vi "Main modul map v3 GPS + kinematyka.vi"() -> ()   [LabVIEW 2012]
uses:
  <vilib>/Utility/miscctls.llb/LVPoint32TypeDef.ctl
  <vilib>/Utility/miscctls.llb/LVBoundsTypeDef.ctl
  <vilib>/Utility/miscctls.llb/LVPointTypeDef.ctl
  Matematyczne/Matematyczne.lvlib
  <vilib>/addons/Fuzzy Logic/NI_Fuzzy_Logic_API.lvlib
  Pomocnicze/Pomocnicze.lvlib
panel:
  in  "Nowa Odl. od startu[m]":cluster{"X [m]":dbl, "Y [m]":dbl}={"X [m]"=-27.201483053257306, "Y [m]"=-30.40589390754667}
  out "x-y":u32
  in  "Lok. mapy odświeżanej":path=path "C:/Users/User/Desktop/Pliki moduł map off-line 2/auto.JPG"
  out "Prędkości kół":cluster{"prawe [rad/s]":dbl, "lewe [rad/s]":dbl}(graph)
  in  "Pocz. poł.":T1 {"UTM"."N [m]" format="%#_10g"}
  out "Mapa":picture caption="Mapa z wprowadzonym punktem"
  out "Lista współrzędnych":string[][](table)
  in  "Tab Control":T2(tab)
  in  "Azymut robota początkowy":dbl min=0.0 max=360.0
  in  "Lokalizacja mapy terenu":path=path "C:/Users/User/Desktop/pł.JPG"
  in  "Parametry odwzorowania Ziemi (WGS84)":cluster{"a":dbl, "b":dbl}={"a"=6378137.0, "b"=6356752.3142} {"b" format="%#.6g"; "a" format="%#.6g"}
  in  "Położenie na mapie":bool
  in  "Zakres skali":u16(ring)=11 items=["OSM 10m", "OSM 30m", "OSM 50m", "OSM 100m"]
  in  "Skalowanie":T3={"Polozenie 1"={"X"=265, "Y"=265}, "  Wybór \nznacznika"=FALSE, "   Polozenie 2"={"X"=358, "Y"=265}, "   Blokada \nznaczników"=FALSE, "Kolor  znaczników"=16774930, "Grubość \nznaczników"=2, "Wyznaczanie odległości"=enum."Odległość pomiędzy znacznikami", "Współrzędne geograficzne 1"="", "Współrzędne geograficzne 2"="", "Odl. pomiędzy znacznikami [m]"=15.0}
  in  "Zatwierdz ustalony zakres":bool
  in  "Odczyt GPS":bool
  in  "Obsługa punktów":T4 {"Usuń punkt z listy"."Punkt do usunięcia" items=["1"=1, "2"=2]}
  in  "Jazda":bool
  out "Dojazd do punktu":string
  out "Zatrzymanie \n w punkcie":bool
  in  "Położenie robota":bool
  in  "Położenie startu":bool
  in  "zad. promien odlegl.":dbl
  in  "Autonomia":bool
  out "Odległość\n od startu [m]":cluster{"X [m]":dbl, "Y [m]":dbl}
  out "Odczyt GPS":T5 caption="Aktualne położenie" {"Szerokośc geograficzna - GPS" format="%_9f"; "Długość geograficzna - GPS" format="%_9f"; "Położenie \nrobota  UTM"."E [m]" format="%#_10g"; "Położenie \nrobota  UTM"."N [m]" format="%#_12g"}
  in  "Właściwości mapy":T7={"Przesunięcie mapy"={"X"=0, "Y"=0}, "Dł. px[m]"=0.19634281539316645, "Zoom mapy"=1.0, "Wpisane punkty na\nliście współrzędnych"=12271, "Zaznaczony punkt"=15663118, "Układ współrzędnych"=0, "Kierunek ruchu robota"=15663118, "Początkowe położenie robota"=15663118, "Trasa robota"=0, "Ost. zazn. pkt"={"X"=0, "Y"=0}, "Draw Area Size"={"Width"=528, "Height"=564}} {"Zoom mapy" scale=0.2..4.0}
  in  "Mouse down":T8
  in  "stop":bool
  # "Ustawienia dla danych z GPS\nPodstaowe parametry Ziemi dla układu WGS84"
  # "Ustawienia dla kinematyki robota."
  # "Nie można usuwać \npunktów, gdy włączona \njest autonomia"
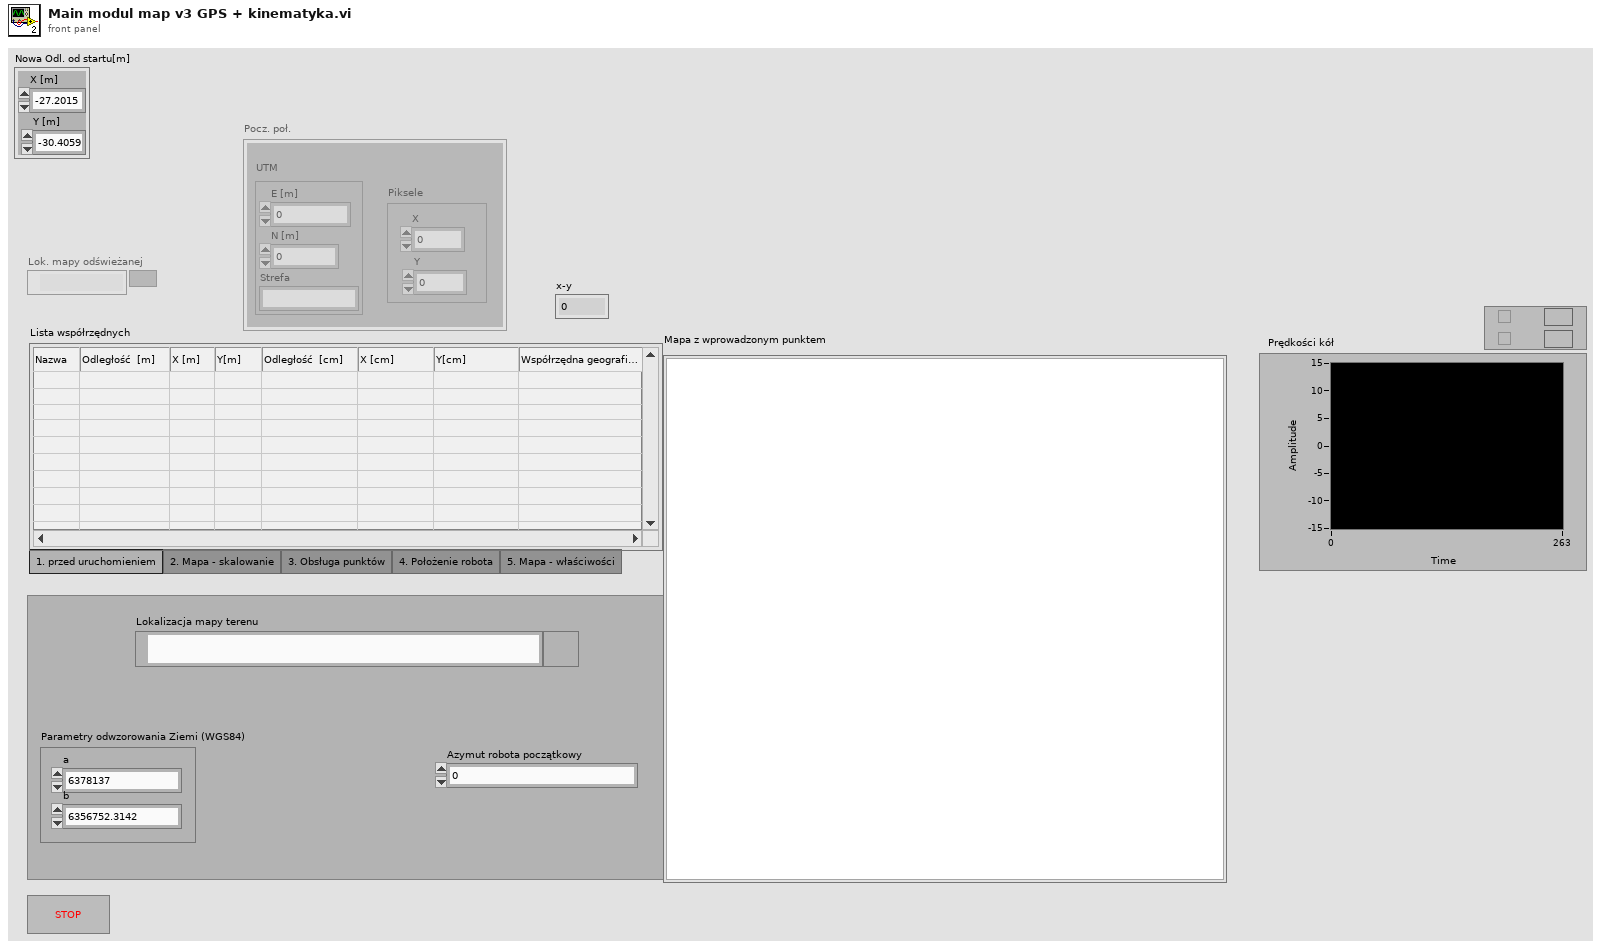
[diagram p1: front panel]
types:
  T1 = cluster{"UTM":cluster{"E [m]":ext, "N [m]":ext, "Strefa":string}, "Piksele":cluster{"X":i32, "Y":i32}}
  T2 = enum32{"1. przed uruchomieniem", "2. Mapa - skalowanie", "3. Obsługa punktów", "4. Położenie robota", "5. Mapa - właściwości"}
  T3 = cluster{"Polozenie 1":cluster{"X":i32, "Y":i32}, "  Wybór \nznacznika":bool, "   Polozenie 2":cluster{"X":i32, "Y":i32}, "   Blokada \nznaczników":bool, "Kolor  znaczników":u32, "Grubość \nznaczników":u32, "Wyznaczanie odległości":enum16{"Współrzędne geograficzne", "Odległość pomiędzy znacznikami"}, "Współrzędne geograficzne 1":string, "Współrzędne geograficzne 2":string, "Odl. pomiędzy znacznikami [m]":dbl}
  T4 = cluster{"Zaznaczony punkt":cluster{"Nazwa":string, "Odl. do pkt [m]":cluster{"X":dbl, "Y":dbl}, "Dodaj punkt odl.":bool}, "Wsp. geograficzne":cluster{"Nazwa":string, "Współrzędna punktu":string, "Dodaj punkt wsp.":bool}, "Usuń punkt z listy":cluster{"Punkt do usunięcia":u16, "Usuń punkt":bool}}
  T5 = cluster{"Położenie \nrobota  UTM":cluster{"E [m]":ext, "N [m]":ext, "Strefa":string}, "Długość geograficzna - GPS":dbl, "Szerokośc geograficzna - GPS":dbl, "Azymut [stopnie]":dbl}
  T6 = typedef "LVBoundsTypeDef.ctl" = cluster{"Width":u32, "Height":u32}
  T7 = cluster{"Przesunięcie mapy":cluster{"X":i16, "Y":i16}, "Dł. px[m]":dbl, "Zoom mapy":sgl, "Wpisane punkty na\nliście współrzędnych":u32, "Zaznaczony punkt":u32, "Układ współrzędnych":u32, "Kierunek ruchu robota":u32, "Początkowe położenie robota":u32, "Trasa robota":u32, "Ost. zazn. pkt":cluster{"X":i32, "Y":i32}, "Draw Area Size":T6}
  T8 = typedef "LVPoint32TypeDef.ctl" = cluster{"Horizontal":i32, "Vertical":i32}
  T9 = enum16{"Pobranie punktu", "Obrót i dojazd do punktu", "Zatrzymanie w punkcie"}
  T10 = typedef "NI_Fuzzy_Logic_API.lvlib/FL System.ctl" = cluster{"input variables":T11[], "output variables":T11[], "rules":T14[], "defuzzification method":T20, "description":string, "user MF interpolating polynomials":T21[]}
  T11 = typedef "NI_Fuzzy_Logic_API.lvlib/FL Variable.ctl" = cluster{"name":string, "range":dbl[], "MFs":T12[]}
  T12 = typedef "NI_Fuzzy_Logic_API.lvlib/FL Membership Function.ctl" = cluster{"name":string, "shape":T13, "points":dbl[], "color":u32, "user-defined shape index":i32}
  T13 = typedef "NI_Fuzzy_Logic_API.lvlib/FL Membership Function Shape.ctl" = u16
  T14 = typedef "NI_Fuzzy_Logic_API.lvlib/FL Rule.ctl" = cluster{"antecedents":T15[], "antecedent connective":T17, "consequents":T18[], "consequent implication":T19, "degree of support":dbl}
  T15 = typedef "NI_Fuzzy_Logic_API.lvlib/FL Antecedent.ctl" = cluster{"Var Index":i32, "MF Index":i32, "Cond":T16}
  T16 = typedef "NI_Fuzzy_Logic_API.lvlib/FL Modifier.ctl" = u16
  T17 = typedef "NI_Fuzzy_Logic_API.lvlib/FL Antecedent Connective.ctl" = u16
  T18 = typedef "NI_Fuzzy_Logic_API.lvlib/FL Consequent.ctl" = cluster{"Var Index":i32, "MF Index":i32, "Cond":T16}
  T19 = typedef "NI_Fuzzy_Logic_API.lvlib/FL Consequent Implication.ctl" = u16
  T20 = typedef "NI_Fuzzy_Logic_API.lvlib/FL Defuzzification.ctl" = u16
  T21 = typedef "NI_Fuzzy_Logic_API.lvlib/FL Interpolating polynomials.ctl" = cluster{"X":dbl[], "Y":dbl[], "Y(x) coeff":dbl[][], "X(y) coeff":dbl[][], "Area(y) coeff":dbl[][], "coa_x(y) coeff":dbl[][]}
  T22 = cluster{"left":i16, "top":i16, "right":i16, "bottom":i16}
  T23 = cluster{"Odl. robota od startu [m]":cluster{"X":dbl, "Y":dbl}, "Położenie startowe":cluster{"X":i32, "Y":i32}, "Azymut [stopnie]":dbl}
  T24 = cluster{"Rozmiar mapy":cluster{"Szerokość":i16, "Wysokość":i16}, "Dł. piksela [m]":dbl, "Trasa robota":u32, "Poł. startowe\n piksele":cluster{"X":i32, "Y":i32}}
  T25 = cluster{"Położenie":cluster{"Pixel x":i16, "Pixel y":i16}, "Kolor punktu":u32, "Rozmiar punktu":u32, "Nazwa punktu":string}
  T26 = cluster{"Kolor punktów z listy":u32, "Położenie startowe robota":cluster{"Pixel y":i16, "Pixel x":i16}}
  T27 = typedef "LVPointTypeDef.ctl" = cluster{"Horizontal":i16, "Vertical":i16}
  T28 = cluster{"Przesunięcie mapy":cluster{"X":i16, "Y":i16}, "Długość piksela w metrach":dbl, "Zoom mapy":sgl, "Wpisane punkty na\nliście współrzędnych":u32, "Zaznaczony punkt":u32, "Układ współrzędnych":u32, "Kierunek ruchu robota":u32, "Początkowe położenie robota":u32, "Trasa robota":u32, "Ostatni zaznaczony punkt na mapie":cluster{"X":i32, "Y":i32}, "Draw Area Size":T6}
  T29 = typedef "LVMouseTypeDef.ctl" = cluster{"Mouse Position":cluster{"X":i32, "Y":i32}, "Mouse Modifiers":cluster{"Button Down":bool, "Shift Mod":bool, "Menu Mod":bool, "Option Mod":bool}}
  T30 = cluster{"Przesunięcie mapy":cluster{"X":i16, "Y":i16}, "Długość piksela w metrach":dbl, "Zoom mapy":sgl, "Wpisane punkty na\nliście współrzędnych":u32, "Zaznaczony punkt":u32, "Układ współrzędnych":u32, "Kierunek ruchu robota":u32, "Początkowe położenie robota":u32, "Trasa robota":u32, "Ost. zazn. pkt.":cluster{"X":i32, "Y":i32}, "Draw Area Size":T6}
  T31 = cluster{"Zaznaczony punkt":cluster{"Nazwa":string, "Odleglosc do\n zaznaczonego punktu [m]":cluster{"X":dbl, "Y":dbl}, "Dodaj punkt odl.":bool}, "Wsp. geograficzne":cluster{"Nazwa":string, "Współrzędna punktu":string, "Dodaj punkt wsp.":bool}, "Usuń punkt z listy":cluster{"Punkt do usunięcia":u16, "Usuń punkt":bool}}
  T32 = cluster{"E [m]":ext, "N [m]":ext, "Strefa":string}
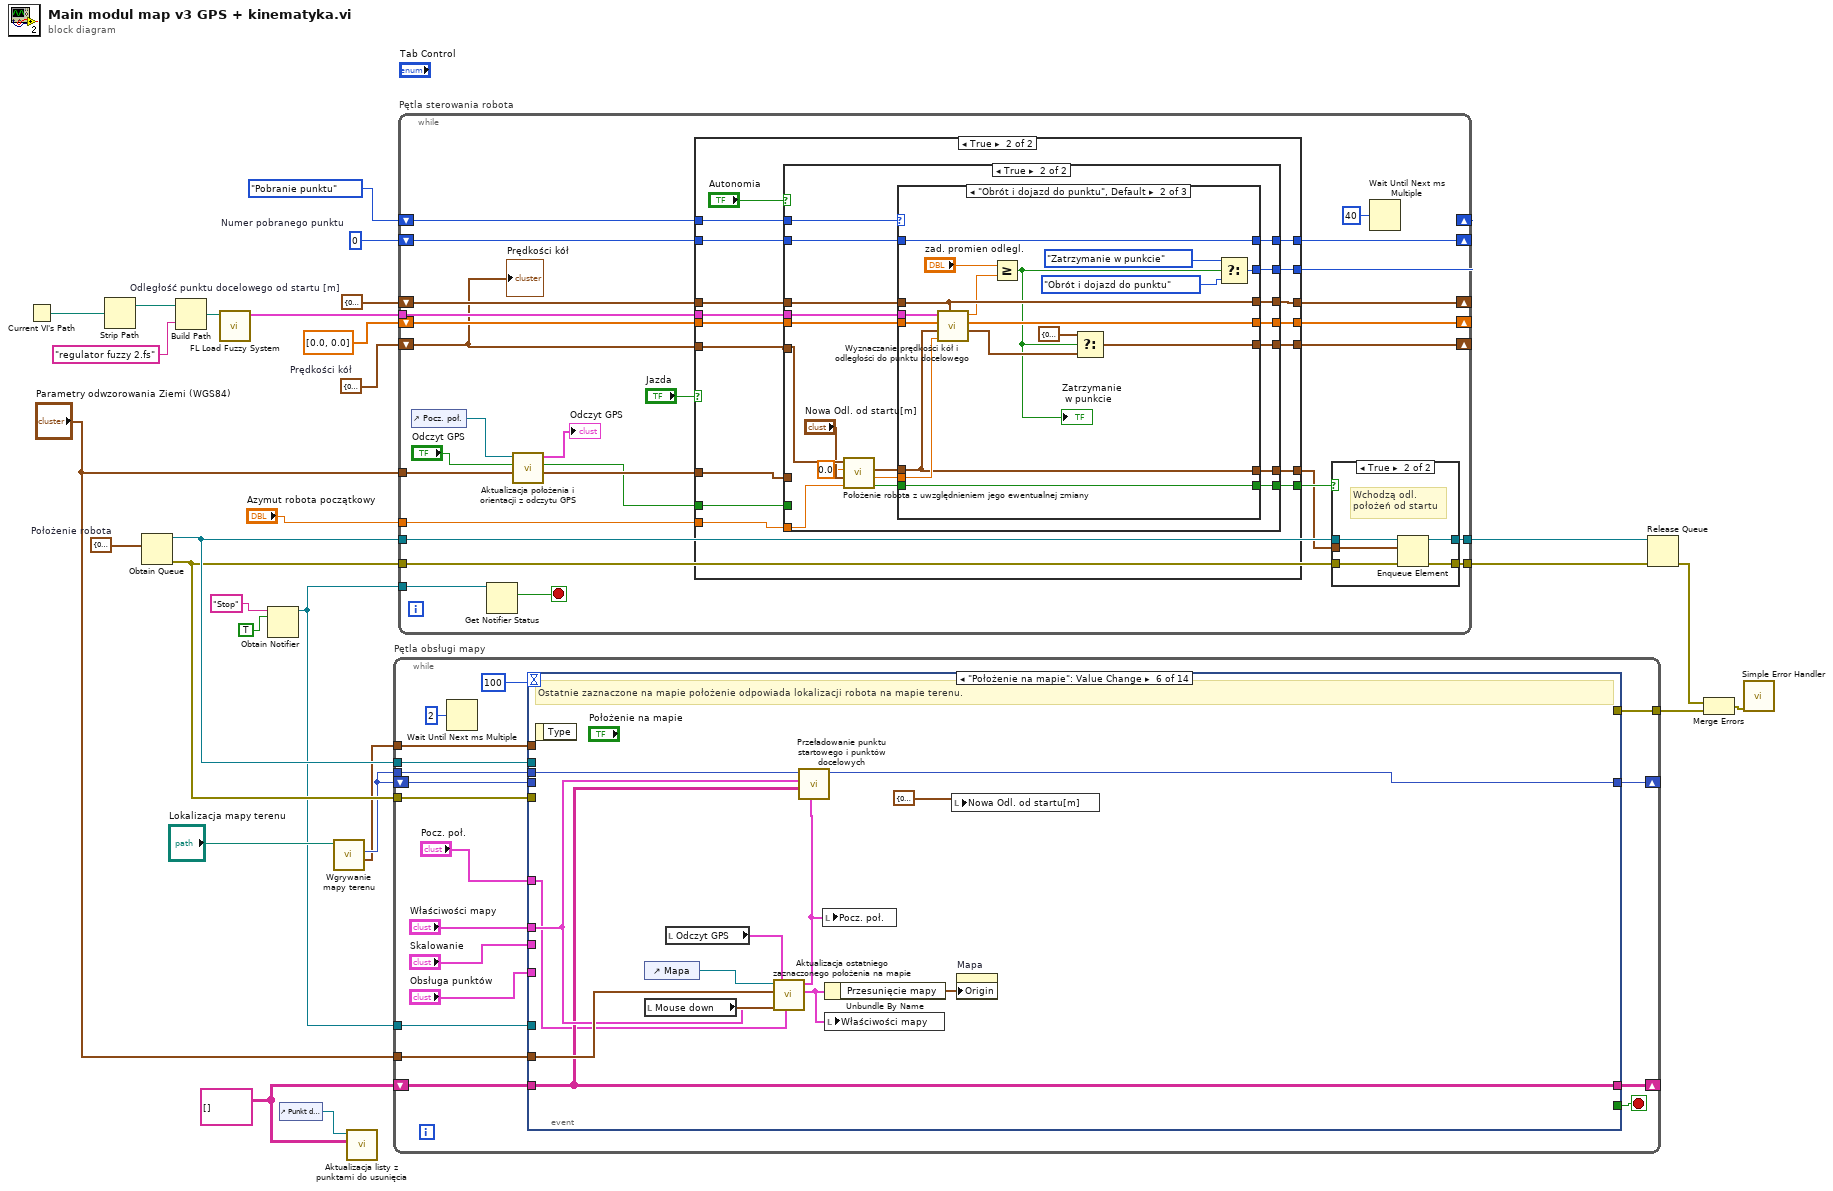
[diagram p0: block diagram]
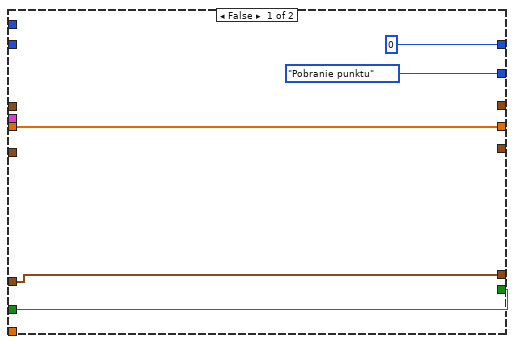
[diagram p3: hidden frame]
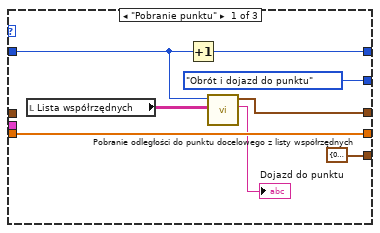
[diagram p4: hidden frame]
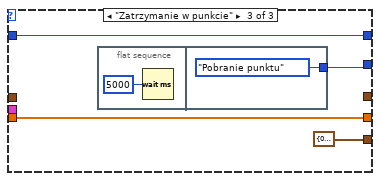
[diagram p5: hidden frame]
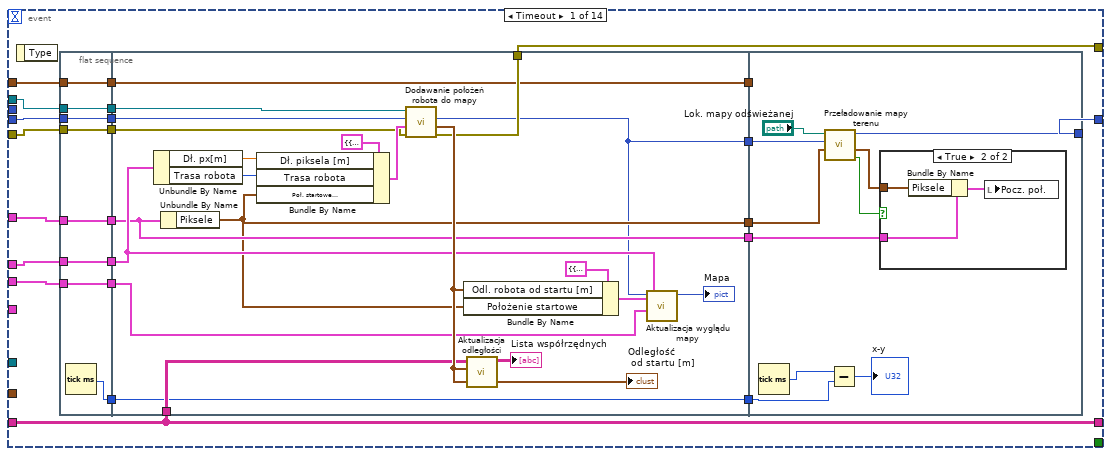
[diagram p7: hidden frame]
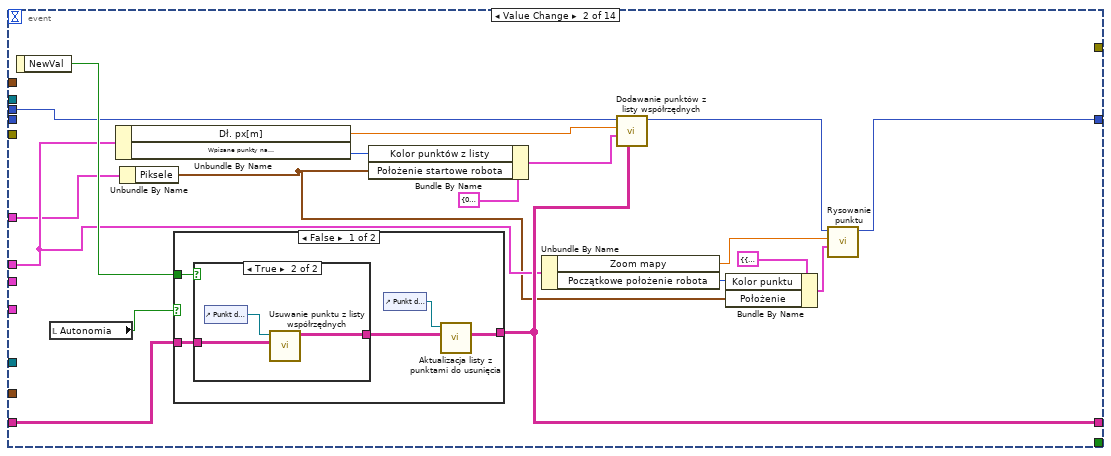
[diagram p9: hidden frame]
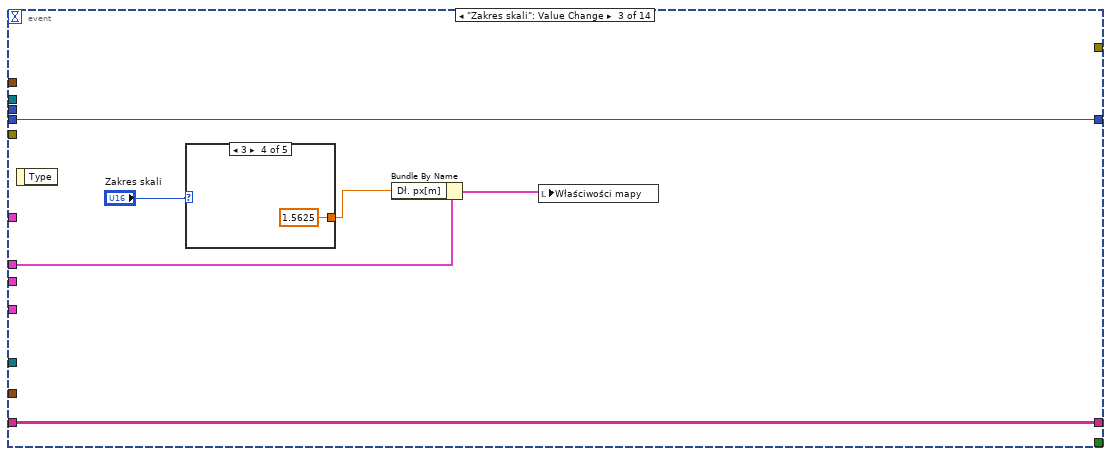
[diagram p12: hidden frame]
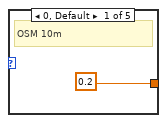
[diagram p13: hidden frame]
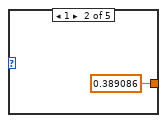
[diagram p14: hidden frame]
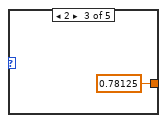
[diagram p15: hidden frame]
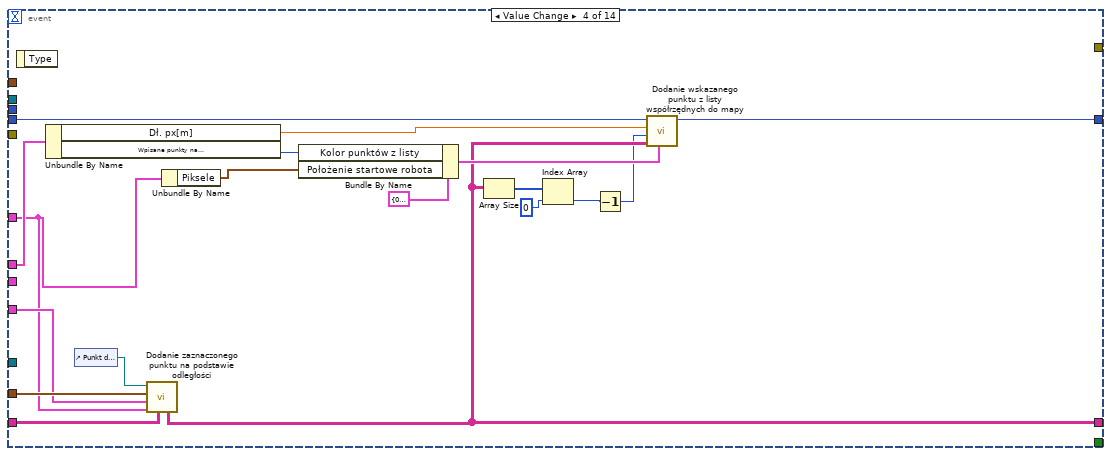
[diagram p17: hidden frame]
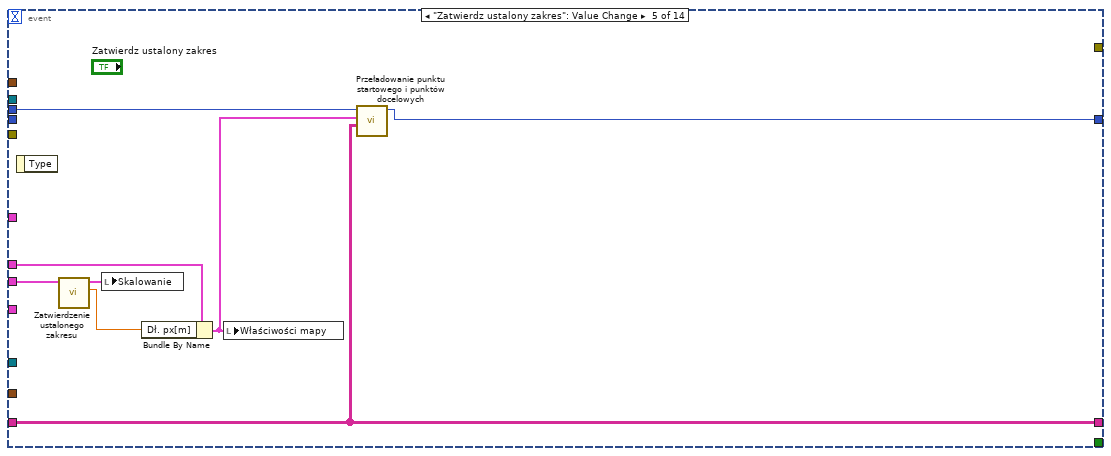
[diagram p18: hidden frame]
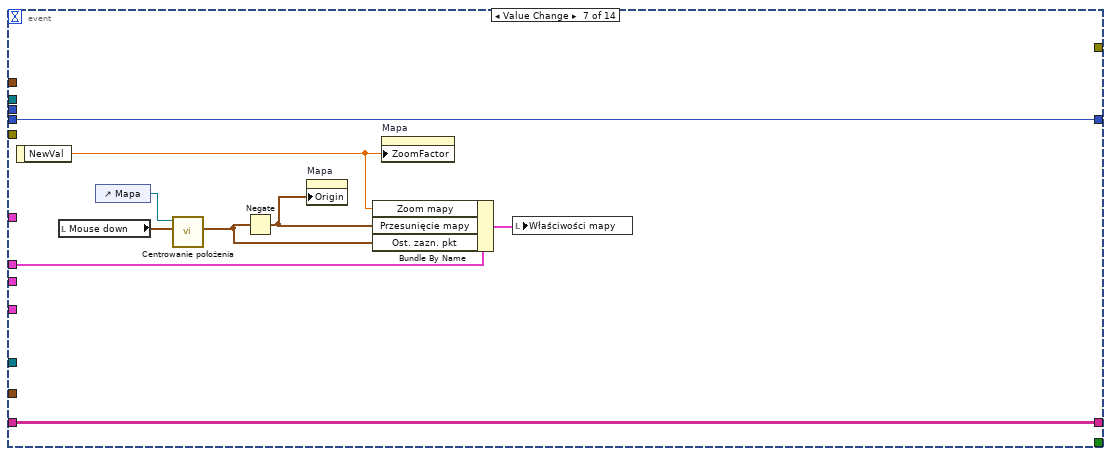
[diagram p19: hidden frame]
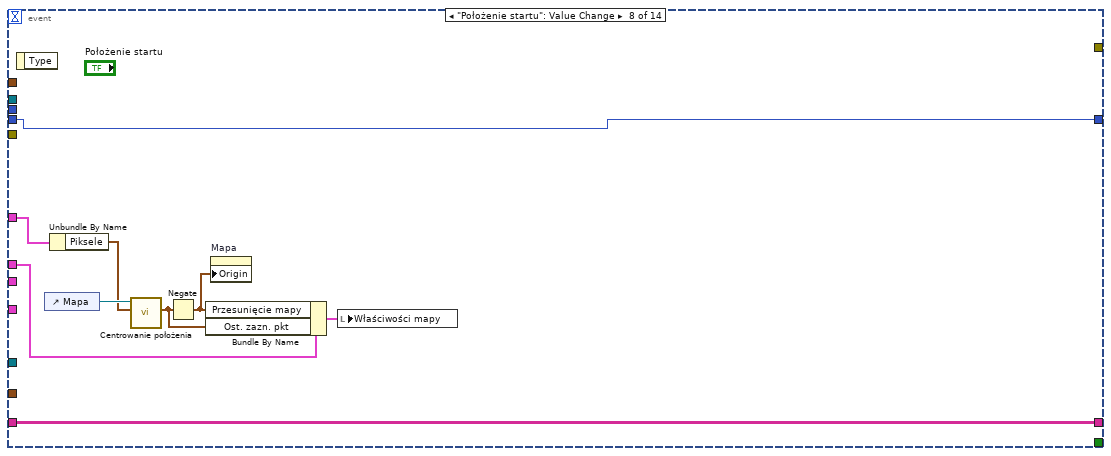
[diagram p20: hidden frame]
diagram:
  w6 = cluster{"prawe [rad/s]":dbl, "lewe [rad/s]":dbl} {"prawe [rad/s]"=0.0, "lewe [rad/s]"=0.0}  # Prędkości kół
  w13 = cluster{"X [m]":dbl, "Y [m]":dbl} {"X [m]"=0.0, "Y [m]"=0.0}  # Położenie robota
  w28 = string[][] [] ("Lista współrzędnych")
  w18 = cluster{"X/E [m]":dbl, "Y/N [m]":dbl} {"X/E [m]"=0.0, "Y/N [m]"=0.0}  # Odległość punktu docelowego od startu [m]
  w19 = 0  # Numer pobranego punktu
  n1 = Current VI's Path() -> (path=w25:path)
  n2 = Strip Path(path=w25) -> (stripped path=w23:path)  [unwired: 1 out]
  n3 = Obtain Queue(element data type=w13) -> (queue out=w10:refnum<queue>, error out=w9:errorcluster)  [unwired: 4 in, 1 out]
  n4 = Build Path(base path=w23, name or relative path="regulator fuzzy 2.fs") -> (appended path=w22:path)
  n5 = call <vilib>:"FL Load Fuzzy System.vi"("file path"=w22) -> ("fuzzy system out"=w21:T10)  [unwired: 1 in, 9 out]
  n6 = Obtain Notifier(name (unnamed)="Stop", notification data type=TRUE ("create if not found? (T)")) -> (notifier out=w4:refnum<notifier>)  [unwired: 2 in, 2 out]
  n7 = control-ref of="Punkt do usunięcia"() -> (w15:refnum<vi>)
  n8 = call "Wgrywanie mapy terenu.vi"("Lokalizacja mapy terenu"="Lokalizacja mapy terenu") -> ("Rozmiar mapy"=w2:T22, "Mapa terenu"=w5:picture)  [unwired: 9 in]
  n9 = call "Aktualizacja listy z punktami do usunięcia.vi"("Lista współrzędnych"=w28, "Lista z punktami do usunięcia"=w15) -> ()  [unwired: 10 in]
  n10 = while "Pętla obsługi mapy" {
    shift-right: [w43] -> _
    shift-left: w5 -> [w44]
    shift-right: [w41] -> _
    shift-left: w28 -> [w42]
    tunnel: "Parametry odwzorowania Ziemi (WGS84)" -> [w40]
    tunnel: w4 -> [w39]
    tunnel: w10 -> [w38]
    tunnel: w9 -> [w33]
    tunnel: w5 -> [w32]
    tunnel: [w31] -> w3
    tunnel: w2 -> [w30]
    stop <- w46 stop-if-true
    n11 = Wait Until Next ms Multiple(millisecond multiple=u32 2) -> ()  [unwired: 1 out]
    n12 = event shown="[5] \"Położenie na mapie\": Value Change" {
      selector: _ -> [_ _ _ _ _ _ _ _ _ _ _ _ _ _]
      dyn-events: _ -> [_ _ _ _ _ _ _ _ _ _ _ _ _ _]
      timeout: 100 -> [_ _ _ _ _ _ _ _ _ _ _ _ _ _]
      tunnel: "Właściwości mapy" -> [w68 w115 w141 w161 w171 w180 w189 w201 w212 w228 _ w247 w267 w286]
      tunnel: w44 -> [w65 _ w144 w154 _ _ w196 w198 w218 w231 w235 w249 w275 w280]
      tunnel: [_ _ _ _ _ _ _ _ _ "stop" _ _ _ _] -> w46
      tunnel: [w61 w113 w144 w150 w167 w178 w196 w198 w218 w231 w235 w249 w275 w277] -> w43
      tunnel: w42 -> [w66 w128 w143 w163 w168 w179 w195 w199 w217 w230 w234 w248 w274 w295]
      tunnel: [w66 w122 w143 w155 w168 w179 w195 w199 w217 w230 w234 w248 w274 w283] -> w41
      tunnel: w40 -> [_ _ _ w166 _ w186 _ _ _ _ _ _ _ _]
      tunnel: w39 -> [_ _ _ _ _ _ _ _ _ w229 _ _ _ _]
      tunnel: w38 -> [w64 _ _ _ _ _ _ _ _ _ _ _ _ _]
      tunnel: "Pocz. poł." -> [w58 w112 _ w149 _ w176 _ w197 w206 _ _ w236 w260 w276]
      tunnel: "Skalowanie" -> [w67 _ _ _ w174 _ _ _ _ _ _ w238 _ _]
      tunnel: "Obsługa punktów" -> [_ _ _ w164 _ _ _ _ _ _ _ w245 w263 w290]
      tunnel: w33 -> [w63 _ _ _ _ _ _ _ _ _ _ _ _ _]
      tunnel: w32 -> [_ w125 _ _ w170 w181 _ _ _ _ _ _ _ _]
      tunnel: [w62 _ _ _ _ _ _ _ _ _ _ _ _ _] -> w31
      tunnel: w30 -> [w59 _ _ _ _ _ _ _ _ _ _ _ _ _]
      event Timeout {
        n13 = event-data() -> ()  [unwired: 1 in, 1 out]
        n14 = flat-sequence {
          tunnel: w58 -> [w71]
          tunnel: w59 -> [w72]
          tunnel: w63 -> [w73]
          tunnel: w64 -> [w74]
          tunnel: w65 -> [w75]
          tunnel: w67 -> [w76]
          tunnel: w68 -> [w77]
          tunnel: [w77] -> w55
          tunnel: [w76] -> w54
          tunnel: [w75] -> w53
          tunnel: [w74] -> w52
          tunnel: [w73] -> w51
          tunnel: [w72] -> w50
          tunnel: [w71] -> w49
          tunnel: [w70] -> w48
          tunnel: [w79] -> w69
          tunnel: w66 -> [w88]
          tunnel: [w84] -> w62
          tunnel: [w83] -> w60
          tunnel: [w80] -> w57
          tunnel: [w81] -> w56
          tunnel: w55 -> [w82]
          tunnel: w54 -> [w89]
          tunnel: w53 -> [w87]
          tunnel: w52 -> [w86]
          tunnel: w51 -> [w85]
          tunnel: w50 -> [w83]
          tunnel: w49 -> [w81]
          tunnel: w48 -> [w78]
          tunnel: [w78] -> w47
          tunnel: [w108] -> w61
          tunnel: w69 -> [w107]
          tunnel: w60 -> [_]
          tunnel: w57 -> [w106]
          tunnel: w56 -> [w102]
          tunnel: w47 -> [w100]
          frame #0 {
            n15 = Tick Count (ms)() -> (millisecond timer value=w70:u32)
          }
          frame #1 {
            n16 = Unbundle By Name(w82) -> ("Dł. px[m]"=w94:dbl, "Trasa robota"=w95:u32)
            n17 = Unbundle By Name(w81) -> ("Piksele"=w80:cluster{"X":i32, "Y":i32})
            n18 = Bundle By Name(cluster=T24 {"Rozmiar mapy"={"Szerokość"=0, "Wysokość"=0}, "Dł. piksela [m]"=0.19634281539316645, "Trasa robota"=16722479, "Poł. startowe\n piksele"={"X"=0, "Y"=0}} ("Dane do wyzn. poł. robota na mapie 2"), "Dł. piksela [m]"=w94, "Trasa robota"=w95, "Poł. startowe\n piksele"=w80) -> (w98:T24)
            n19 = call "Dodawanie położeń robota do mapy.vi"("error in (no error)"=w85, "Dane do wyzn. poł. robota na mapie"=w98, "Mapa terenu"=w87, "Dane z położenia"=w86) -> ("error out"=w84:errorcluster, "Odległość robota od startu [m]"=w97:cluster{"X [m]":dbl, "Y [m]":dbl}, "Mapa z wprowadzonym punktem"=w79:picture)  [unwired: 5 in]
            "Odległość\n od startu [m]" <- w97
            n20 = Bundle By Name(cluster=T23 {"Odl. robota od startu [m]"={"X"=246.0, "Y"=243.0}, "Położenie startowe"={"X"=246, "Y"=243}, "Azymut [stopnie]"=297.94899101038743} ("Położenie robota"), "Odl. robota od startu [m]"=w97, "Położenie startowe"=w80) -> (w96:T23)
            n21 = call "Aktualizacja odległości.vi"("Odległość od startu [m]"=w97, "Lista współrzędnych"=w88) -> ("Lista współrzędnych 2"=→"Lista współrzędnych":string[][])  [unwired: 9 in]
            n22 = call "Aktualizacja wyglądu mapy.vi"("Położenie robota"=w96, "Skalowanie i kolory"=w89, "Właściwości mapy"=w82, "Mapa"=w79) -> ("Przesunięta mapa"=→"Mapa":picture)  [unwired: 7 in]
          }
          frame #2 {
            n23 = Tick Count (ms)() -> (millisecond timer value=w101:u32)
            n24 = call "Przeładowanie mapy terenu.vi"("Położenie startowe"=w106, ">mapa z trasą robota>"=w107, "path to JPEG file"="Lok. mapy odświeżanej") -> ("reload"=w105:bool, "Nowe położenie  startowe [px]"=w103:cluster{"X [px]":i16, "Y [px]":i16}, "Mapa terenu"=w108:picture)  [unwired: 6 in]
            n25 = Subtract(x=w101, y=w100) -> (x-y=→"x-y":u32)
            n26 = case shown="True" w105 {
              tunnel: w103 -> [_ w111]
              tunnel: w102 -> [_ w110]
              frame False {
              }
              frame True {
                n27 = Bundle By Name(cluster=w110, "Piksele"=w111) -> (w109:T1)
                n28 = local write "Pocz. poł."(w109) -> ()
              }
            }
          }
        }
      }
      event "Obsługa punktów.Usuń punkt z listy.Usuń punkt": Value Change {
        n29 = event-data() -> ("NewVal"=w129:bool)  [unwired: 1 in]
        n30 = local read "Autonomia"() -> (w127:bool)
        n31 = Unbundle By Name(w115) -> ("Dł. px[m]"=w124:dbl, "Wpisane punkty na\nliście współrzędnych"=w126:u32)
        n32 = Unbundle By Name(w112) -> ("Piksele"=w114:cluster{"X":i32, "Y":i32})
        n33 = case shown="False" w127 {
          tunnel: w129 -> [w133 _]
          tunnel: w128 -> [w131 w138]
          tunnel: [w130 w138] -> w122
          frame False {
            n34 = case shown="True" w133 {
              tunnel: w131 -> [w134 w136]
              tunnel: [w134 w135] -> w130
              frame False {
              }
              frame True {
                n35 = control-ref of="Punkt do usunięcia"() -> (w137:refnum<vi>)
                n36 = call "Usuwanie punktu z listy współrzędnych.vi"("Lista współrzędnych"=w136, "Lista z punktami do usunięcia"=w137) -> ("Lista współrzędnych 2"=w135:string[][])  [unwired: 9 in]
              }
            }
            n37 = control-ref of="Punkt do usunięcia"() -> (w132:refnum<vi>)
            n38 = call "Aktualizacja listy z punktami do usunięcia.vi"("Lista współrzędnych"=w130, "Lista z punktami do usunięcia"=w132) -> ()  [unwired: 10 in]
          }
          frame True {
          }
        }
        n39 = Bundle By Name(cluster=T26 {"Kolor punktów z listy"=0, "Położenie startowe robota"={"Pixel y"=0, "Pixel x"=0}} ("Właściwości punktów z listy"), "Kolor punktów z listy"=w126, "Położenie startowe robota"=w114) -> (w121:T26)
        n40 = Unbundle By Name(w115) -> ("Zoom mapy"=w118:sgl, "Początkowe położenie robota"=w117:u32)
        n41 = call "Dodawanie punktów z listy współrzędnych.vi"("Lista współrzędnych"=w122, "Właściwości punktów z listy"=w121, "Długość piksela w metrach"=w124, "Mapa terenu"=w125) -> ("Mapa z wprowadzonym punktem"=w116:picture)  [unwired: 6 in, 1 out]
        n42 = Bundle By Name(cluster=T25 {"Położenie"={"Pixel x"=246, "Pixel y"=243}, "Kolor punktu"=15663118, "Rozmiar punktu"=2, "Nazwa punktu"=""} ("Punkt na mapie"), "Kolor punktu"=w117, "Położenie"=w114) -> (w119:T25)
        n43 = call "Rysowanie punktu.vi"("Punkt na mapie"=w119, "Zoom mapy"=w118, "Mapa terenu"=w116) -> ("Mapa z wprowadzonym punktem"=w113:picture)  [unwired: 8 in]
      }
      event "Zakres skali": Value Change {
        n44 = event-data() -> ()  [unwired: 1 in, 1 out]
        n45 = case shown="3" "Zakres skali" {
          tunnel: [0.2 0.389086 0.78125 1.5625 _] -> w139
          frame 0, Default {
            # "OSM 10m"
          }
          frame 1 {
          }
          frame 2 {
          }
          frame 3 {
          }
          frame 4 {
          }
        }
        n46 = Bundle By Name(cluster=w141, "Dł. px[m]"=w139) -> (w140:T7)
        n47 = local write "Właściwości mapy"(w140) -> ()
      }
      event "Obsługa punktów.Zaznaczony punkt.Dodaj punkt odl.": Value Change {
        n48 = event-data() -> ()  [unwired: 1 in, 1 out]
        n49 = Unbundle By Name(w161) -> ("Dł. px[m]"=w157:dbl, "Wpisane punkty na\nliście współrzędnych"=w160:u32)
        n50 = control-ref of="Punkt do usunięcia"() -> (w165:refnum<vi>)
        n51 = call "Dodanie zaznaczonego punktu na podstawie odległości.vi"("output array in"=w163, "Pocz. poł."=w149, "Obsługa punktów"=w164, "Parametry odwzorowania Ziemi (WGS84)"=w166, "Ring in"=w165) -> ("output array out"=w155:string[][])  [unwired: 6 in]
        n52 = Unbundle By Name(w149) -> ("Piksele"=w151:cluster{"X":i32, "Y":i32})
        n53 = Bundle By Name(cluster=T26 {"Kolor punktów z listy"=0, "Położenie startowe robota"={"Pixel y"=0, "Pixel x"=0}} ("Właściwości punktów z listy"), "Kolor punktów z listy"=w160, "Położenie startowe robota"=w151) -> (w156:T26)
        n54 = Array Size(array=w155) -> (size(s)=w158:i32[])
        n55 = Index Array(array=w158, index=0) -> (element=w153:i32)
        n56 = Decrement(x=w153) -> (x-1=w152:i32)
        n57 = call "Dodanie wskazanego punktu z listy współrzędnych do mapy.vi"("Właściwości punktów z listy"=w156, "Lista współrzędnych"=w155, "Nr punktu"=w152, "Długość piksela w metrach"=w157, "Mapa terenu"=w154) -> ("Mapa z wprowadzonym punktem"=w150:picture)  [unwired: 5 in, 1 out]
      }
      event "Zatwierdz ustalony zakres": Value Change {
        n58 = event-data() -> ()  [unwired: 1 in, 1 out]
        n59 = call "Zatwierdzenie ustalonego zakresu.vi"("Skalowanie in"=w174) -> ("Dł. piksela[m]"=w172:dbl, "Skalowanie out"=w173:T3)  [unwired: 9 in]
        n60 = local write "Skalowanie"(w173) -> ()
        n61 = Bundle By Name(cluster=w171, "Dł. px[m]"=w172) -> (w169:T7)
        n62 = local write "Właściwości mapy"(w169) -> ()
        n63 = call "Przeładowanie punktu startowego i punktów docelowych.vi"("Lista współrzędnych"=w168, "Właściwości mapy"=w169, "Mapa terenu"=w170) -> ("Mapa z wprowadzonym punktem"=w167:picture)  [unwired: 8 in]
      }
      event "Położenie na mapie": Value Change {
        # "Ostatnie zaznaczone na mapie położenie odpowiada lokalizacji robota na mapie terenu."
        n64 = event-data() -> ()  [unwired: 1 in, 1 out]
        n65 = control-ref of="Mapa"() -> (w185:refnum<vi>)
        n66 = local read "Mouse down"() -> (w187:T8)
        n67 = local read "Odczyt GPS"() -> (w182:T5)
        n68 = call "Aktualizacja ostatniego zaznaczonego położenia na mapie.vi"("Pocz. poł."=w176, "Aktualne położenie"=w182, "Właściwości mapy in"=w180, "Mouse down coords"=w187, "Parametry odwzorowania Ziemi (WGS84)"=w186, "Picture in"=w185) -> ("Właściwości mapy out"=w184:T28, "Pocz. poł. 2"=w177:T1)  [unwired: 4 in]
        n69 = call "Przeładowanie punktu startowego i punktów docelowych.vi"("Pocz. poł. in"=w177, "Lista współrzędnych"=w179, "Właściwości mapy"=w180, "Mapa terenu"=w181) -> ("Mapa z wprowadzonym punktem"=w178:picture)  [unwired: 7 in]
        n70 = local write "Pocz. poł."(w177) -> ()
        n71 = Unbundle By Name(w184) -> ("Przesunięcie mapy"=w183:cluster{"X":i16, "Y":i16})
        n72 = local write "Właściwości mapy"(w184) -> ()
        n73 = local write "Nowa Odl. od startu[m]"(cluster{"X [m]":dbl, "Y [m]":dbl} {"X [m]"=0.0, "Y [m]"=0.0} ("Nowa Odl. od startu[m]")) -> ()
        n74 = property on="Mapa" class="Pict"("Origin"=w183) -> ()  [unwired: 2 in, 2 out]
      }
      event "Właściwości mapy.Zoom mapy": Value Change {
        n75 = event-data() -> ("NewVal"=w193:sgl)  [unwired: 1 in]
        n76 = local read "Mouse down"() -> (w188:T8)
        n77 = control-ref of="Mapa"() -> (w194:refnum<vi>)
        n78 = call "Centrowanie położenia.vi"("Ostatnie położenie robota"=w188, "Mapa z wprowadzonym punktem"=w194) -> ("Przesunięcie wycentrowane"=w191:T8)  [unwired: 9 in]
        n79 = Negate(x=w191) -> (-x=w190:T8)
        n80 = property on="Mapa" class="Pict"("Origin"=w190) -> ()  [unwired: 2 in, 2 out]
        n81 = Bundle By Name(cluster=w189, "Zoom mapy"=w193, "Przesunięcie mapy"=w190, "Ost. zazn. pkt"=w191) -> (w192:T7)
        n82 = property on="Mapa" class="Pict"("ZoomFactor"=w193) -> ()  [unwired: 2 in, 2 out]
        n83 = local write "Właściwości mapy"(w192) -> ()
      }
      event "Położenie startu": Value Change {
        n84 = event-data() -> ()  [unwired: 1 in, 1 out]
        n85 = control-ref of="Mapa"() -> (w205:refnum<vi>)
        n86 = Unbundle By Name(w197) -> ("Piksele"=w200:cluster{"X":i32, "Y":i32})
        n87 = call "Centrowanie położenia.vi"("Ostatnie położenie robota"=w200, "Mapa z wprowadzonym punktem"=w205) -> ("Przesunięcie wycentrowane"=w203:T8)  [unwired: 9 in]
        n88 = Negate(x=w203) -> (-x=w202:T8)
        n89 = Bundle By Name(cluster=w201, "Przesunięcie mapy"=w202, "Ost. zazn. pkt"=w203) -> (w204:T7)
        n90 = property on="Mapa" class="Pict"("Origin"=w202) -> ()  [unwired: 2 in, 2 out]
        n91 = local write "Właściwości mapy"(w204) -> ()
      }
      event "Położenie robota": Value Change {
        n92 = event-data() -> ()  [unwired: 1 in, 1 out]
        n93 = local read "Odległość\n od startu [m]"() -> (w211:cluster{"X [m]":dbl, "Y [m]":dbl})
        n94 = Unbundle By Name(w212) -> ("Dł. px[m]"=w210:dbl)
        n95 = Unbundle By Name(w206) -> ("Piksele"=w208:cluster{"X":i32, "Y":i32})
        n96 = in-place {
          in-place-border: w210 -> [w221]
          n97 = in-place-cluster #1(w211) -> ("X [m]"=w220:dbl, "Y [m]"=w219:dbl)
          n98 = Divide(x=w219, y=w221) -> (x/y=w222:dbl)
          n99 = Divide(x=w220, y=w221) -> (x/y=w224:dbl)
          n100 = Negate(x=w222) -> (-x=w223:dbl)
          n101 = in-place-cluster #1("X [m]"=w224, "Y [m]"=w223) -> (w209:cluster{"X [m]":dbl, "Y [m]":dbl})
        }
        n102 = Add(x=w209, y=w208) -> (x+y=w207:cluster{dbl, dbl})
        n103 = control-ref of="Mapa"() -> (w216:refnum<vi>)
        n104 = call "Centrowanie położenia.vi"("Ostatnie położenie robota"=w207, "Mapa z wprowadzonym punktem"=w216) -> ("Przesunięcie wycentrowane"=w214:T8)  [unwired: 9 in]
        n105 = Negate(x=w214) -> (-x=w213:T8)
        n106 = Bundle By Name(cluster=w212, "Przesunięcie mapy"=w213, "Ost. zazn. pkt"=w214) -> (w215:T7)
        n107 = property on="Mapa" class="Pict"("Origin"=w213) -> ()  [unwired: 2 in, 2 out]
        n108 = local write "Właściwości mapy"(w215) -> ()
      }
      event "stop": Value Change {
        n109 = event-data() -> ()  [unwired: 1 in, 1 out]
        n110 = Bundle By Name(cluster=w228, "Przesunięcie mapy"=T27 {"Horizontal"=0, "Vertical"=0} ("Origin")) -> (w227:T7)
        n111 = local write "Właściwości mapy"(w227) -> ()
        n112 = Send Notification(notification="stop", notifier=w229) -> ()  [unwired: 1 in, 2 out]
      }
      event "Mapa": Mouse Down {
        # "Odczyt lokalizacji kursora po kliknięciu na mapie."
        n113 = event-data() -> ()  [unwired: 1 in, 2 out]
        n114 = property on="Mapa" class="Pict"() -> ("Mouse"=w233:T29)  [unwired: 2 in, 2 out]
        n115 = Unbundle By Name(w233) -> ("Mouse Position"=w232:cluster{"X":i32, "Y":i32})
        n116 = local write "Mouse down"(w232) -> ()
      }
      event "Mapa": Mouse Up {
        # "Wyznaczenie zmiany położenia przed i po kliknięciu."
        n117 = event-data() -> ()  [unwired: 1 in, 1 out]
        n118 = property on="Mapa" class="Pict"() -> ("Mouse"=w246:T29)  [unwired: 2 in, 2 out]
        n119 = call "Ustalenie nowego przesunięcia mapy po mose down-up.vi"("Właściwości mapy in"=w247, "Pocz. poł."=w236, "Obsługa punktów in"=w245, "Mouse down \ncoords"="Mouse down", "Mouse"=w246) -> ("Właściwości mapy out"=w242:T30, "Obsługa punktów out"=w244:T31)  [unwired: 5 in]
        n120 = local write "Obsługa punktów"(w244) -> ()
        n121 = local write "Właściwości mapy"(w242) -> ()
        n122 = Unbundle By Name(w242) -> ("Ost. zazn. pkt."=w237:cluster{"X":i32, "Y":i32}, "Przesunięcie mapy"=w241:cluster{"X":i16, "Y":i16})
        n123 = Unbundle By Name(w238) -> ("Wybór \nznacznika"=w240:bool, "Blokada \nznaczników"=w239:bool)
        n124 = property on="Mapa" class="Pict"("Origin"=w241) -> ()  [unwired: 2 in, 2 out]
        n125 = case shown="False" w239 {
          tunnel: w240 -> [w253 _]
          tunnel: w238 -> [w252 _]
          tunnel: w237 -> [w250 _]
          frame False {
            n126 = case shown="True" w253 {
              tunnel: w252 -> [w256 w259]
              tunnel: [w255 w258] -> w251
              tunnel: w250 -> [w254 w257]
              frame False {
                n127 = Bundle By Name(cluster=w256, "Polozenie 1"=w254) -> (w255:T3)
              }
              frame True {
                n128 = Bundle By Name(cluster=w259, "Polozenie 2"=w257) -> (w258:T3)
              }
            }
            n129 = local write "Skalowanie"(w251) -> ()
          }
          frame True {
          }
        }
      }
      event "Obsługa punktów.Zaznaczony punkt.Odl. do pkt [m]": Value Change {
        n130 = event-data() -> ()  [unwired: 1 in, 1 out]
        n131 = Unbundle By Name(w263) -> ("Zaznaczony punkt.Odl. do pkt [m].X"=w262:dbl, "Zaznaczony punkt.Odl. do pkt [m].Y"=w261:dbl)
        n132 = Unbundle By Name(w260) -> ("Piksele.X"=w269:i32, "Piksele.Y"=w268:i32)
        n133 = Unbundle By Name(w267) -> ("Dł. px[m]"=w273:dbl)
        n134 = Divide(x=w262, y=w273) -> (x/y=w271:dbl)
        n135 = Negate(x=w261) -> (-x=w272:dbl)
        n136 = Divide(x=w272, y=w273) -> (x/y=w270:dbl)
        n137 = Add(x=w271, y=w269) -> (x+y=w266:dbl)
        n138 = Add(x=w270, y=w268) -> (x+y=w265:dbl)
        n139 = Bundle By Name(cluster=w267, "Ost. zazn. pkt.X"=w266, "Ost. zazn. pkt.Y"=w265) -> (w264:T7)
        n140 = local write "Właściwości mapy"(w264) -> ()
      }
      event "Obsługa punktów.Wsp. geograficzne.Dodaj punkt wsp.": Value Change {
        n141 = event-data() -> ()  [unwired: 1 in, 1 out]
        n142 = Unbundle By Name(w286) -> ("Dł. px[m]"=w282:dbl, "Wpisane punkty na\nliście współrzędnych"=w288:u32)
        n143 = Unbundle By Name(w290) -> ("Wsp. geograficzne.Nazwa"=w292:string, "Wsp. geograficzne.Współrzędna punktu"=w291:string)
        n144 = Unbundle By Name(w276) -> ("UTM"=w293:T32)
        n145 = Unbundle By Name(w276) -> ("Piksele"=w287:cluster{"X":i32, "Y":i32})
        n146 = Bundle By Name(cluster=T26 {"Kolor punktów z listy"=0, "Położenie startowe robota"={"Pixel y"=0, "Pixel x"=0}} ("Właściwości punktów z listy"), "Kolor punktów z listy"=w288, "Położenie startowe robota"=w287) -> (w281:T26)
        n147 = call "Dodanie punktu do listy punkty na podstawie współrzędnych geograficznych.vi"("Nazwa punktu"=w292, "UTM"=w293, "Współrzędne punktu"=w291, "Lista wsp. in"=w295) -> ("Lista wsp. out"=w283:string[][])  [unwired: 7 in]
        n148 = control-ref of="Punkt do usunięcia"() -> (w294:refnum<vi>)
        n149 = call "Aktualizacja listy z punktami do usunięcia.vi"("Lista współrzędnych"=w283, "Lista z punktami do usunięcia"=w294) -> ()  [unwired: 10 in]
        n150 = Array Size(array=w283) -> (size(s)=w284:i32[])
        n151 = Index Array(array=w284, index=0) -> (element=w279:i32)
        n152 = Decrement(x=w279) -> (x-1=w278:i32)
        n153 = call "Dodanie wskazanego punktu z listy współrzędnych do mapy.vi"("Właściwości punktów z listy"=w281, "Lista współrzędnych"=w283, "Nr punktu"=w278, "Długość piksela w metrach"=w282, "Mapa terenu"=w280) -> ("Mapa z wprowadzonym punktem"=w277:picture)  [unwired: 5 in, 1 out]
      }
    }
  }
  n154 = while "Pętla sterowania robota" {
    tunnel: w4 -> [w323]
    tunnel: w21 -> [w321]
    shift-right: [w307] -> _
    shift-left: dbl[] [0.0, 0.0] ("input values") -> [w320]
    shift-right: [w316] -> _
    shift-left: T9."Pobranie punktu" -> [w319]
    shift-right: [w317] -> _
    shift-left: w19 -> [w318]
    shift-right: [w315] -> _
    shift-left: w18 -> [w314]
    tunnel: "Parametry odwzorowania Ziemi (WGS84)" -> [w313]
    tunnel: w10 -> [w312]
    tunnel: [w311] -> w12
    tunnel: [w310] -> w11
    tunnel: w9 -> [w309]
    shift-right: [w306] -> _
    shift-left: w6 -> [w302]
    tunnel: "Azymut robota początkowy" -> [w299]
    stop <- w322 stop-if-true
    n155 = control-ref of="Pocz. poł."() -> (w297:refnum<vi>)
    n156 = Get Notifier Status(notifier=w323) -> (current notification=w322:bool)  [unwired: 1 in, 4 out]
    n157 = call "Aktualizacja położenia i orientacji z odczytu GPS.vi"("Parametry odwzorowania Ziemi (WGS84)"=w313, "Odczyt GPS"="Odczyt GPS", "Cluster in"=w297) -> ("Rzeczywista odległość robota od startu [m]"=w305:cluster{"X [m]":dbl, "Y [m]":dbl}, "Time has Elapsed"=w300:bool, "Aktualne położenie"=→"Odczyt GPS":T5)  [unwired: 6 in]
    n158 = case shown="True" "Jazda" {
      tunnel: w321 -> [_ w340]
      tunnel: w320 -> [_ w339]
      tunnel: w319 -> [_ w338]
      tunnel: w318 -> [_ w337]
      tunnel: [_ w336] -> w317
      tunnel: [_ w335] -> w316
      tunnel: [_ w334] -> w315
      tunnel: w314 -> [_ w333]
      tunnel: [_ w331] -> w307
      tunnel: [_ w330] -> w306
      tunnel: w305 -> [_ w329]
      tunnel: [_ w328] -> w304
      tunnel: [_ w327] -> w303
      tunnel: w302 -> [_ w326]
      tunnel: w300 -> [_ w325]
      tunnel: w299 -> [_ w324]
      frame False {
      }
      frame True {
        n159 = case shown="True" "Autonomia" {
          tunnel: w340 -> [_ w364]
          tunnel: w339 -> [w345 w363]
          tunnel: [w345 w362] -> w331
          tunnel: w338 -> [_ w361]
          tunnel: w337 -> [_ w360]
          tunnel: [0 ("Numer pobranego punktu") w359] -> w336
          tunnel: [T9."Pobranie punktu" w358] -> w335
          tunnel: [_ w357] -> w334
          tunnel: w333 -> [_ w356]
          tunnel: w326 -> [_ w353]
          tunnel: [_ w352] -> w330
          tunnel: w329 -> [w342 _]
          tunnel: [w341 w350] -> w328
          tunnel: [w342 w349] -> w327
          tunnel: w325 -> [w341 _]
          tunnel: w324 -> [_ w348]
          frame False {
          }
          frame True {
            n160 = call "Położenie robota z uwzględnieniem jego ewentualnej zmiany.vi"("Azymut startowy"=w348, "Nowa Odl. od startu[m]"="Nowa Odl. od startu[m]", "Azymut robota"=0.0, "Prędkości kół"=w353) -> ("Zmiana położenia robota?"=w354:bool, "Azymut [stopnie]"=w355:dbl, "Odległość robota od startu"=w351:cluster{"X[m]":dbl, "Y[m]":dbl})  [unwired: 5 in]
            n161 = case shown="\"Obrót i dojazd do punktu\", Default" w361 {
              tunnel: w364 -> [_ w384 _]
              tunnel: w363 -> [w368 w383 w392]
              tunnel: [w368 w389 w392] -> w362
              tunnel: w360 -> [w369 w385 w393]
              tunnel: [w372 w385 w393] -> w359
              tunnel: [T9."Obrót i dojazd do punktu" w386 w390] -> w358
              tunnel: [w370 w381 _] -> w357
              tunnel: w356 -> [_ w381 _]
              tunnel: w351 -> [_ w379 _]
              tunnel: w355 -> [_ w382 _]
              tunnel: w354 -> [_ w380 _]
              tunnel: [cluster{"prawe [rad/s]":dbl, "lewe [rad/s]":dbl} {"prawe [rad/s]"=0.0, "lewe [rad/s]"=0.0} ("Prędkości kół") w375 cluster{"prawe [rad/s]":dbl, "lewe [rad/s]":dbl} {"prawe [rad/s]"=0.0, "lewe [rad/s]"=0.0} ("Prędkości kół")] -> w352
              tunnel: [_ w380 _] -> w350
              tunnel: [_ w379 _] -> w349
              frame "Pobranie punktu" {
                n162 = local read "Lista współrzędnych"() -> (w367:string[][])
                n163 = Increment(x=w369) -> (x+1=w372:i32)
                n164 = call "Pobranie odległości do punktu docelowego z listy współrzędnych.vi"("Lista współrzędnych"=w367, "Numer pobranego punktu"=w369) -> ("Dojazd do punktu"=→"Dojazd do punktu":string, "Odl. do punktu docelowego"=w370:cluster{"X/E [m]":dbl, "Y/N [m]":dbl})  [unwired: 8 in]
              }
              frame "Obrót i dojazd do punktu", Default {
                n165 = call "Wyznaczanie prędkości kół i odległości do punktu docelowego.vi"("Odl. pkt. docelowego od startu[m]"=w381, "Azymut robota [stopnie]"=w382, "Odległość robota od startu"=w379, "Odległość i odchylenie kątowe"=w383, "fuzzy system in"=w384) -> ("Prędkości kół"=w376:cluster{"prawe [rad/s]":dbl, "lewe [rad/s]":dbl}, "Odległość i odchylenie kątowe"=w389:dbl[], "Odległość do punktu zadanego [m]"=w377:dbl)  [unwired: 4 in]
                n166 = Greater Or Equal?(x="zad. promien odlegl.", y=w377) -> (x >= y?=w373:bool)
                "Zatrzymanie \n w punkcie" <- w373
                n167 = Select(t=cluster{"prawe [rad/s]":dbl, "lewe [rad/s]":dbl} {"prawe [rad/s]"=0.0, "lewe [rad/s]"=0.0}, s=w373, f=w376) -> (s? t:f=w375:cluster{"prawe [rad/s]":dbl, "lewe [rad/s]":dbl})
                n168 = Select(t=T9."Zatrzymanie w punkcie", s=w373, f=T9."Obrót i dojazd do punktu") -> (s? t:f=w386:T9)
              }
              frame "Zatrzymanie w punkcie" {
                n169 = flat-sequence {
                  tunnel: [T9."Pobranie punktu"] -> w390
                  frame #0 {
                    n170 = Wait (ms)(milliseconds to wait=u32 5000) -> ()  [unwired: 1 out]
                  }
                  frame #1 {
                  }
                }
              }
            }
          }
        }
      }
    }
    n171 = case shown="True" w304 {
      tunnel: w312 -> [w397 w402]
      tunnel: [w397 w401] -> w311
      tunnel: [w396 w400] -> w310
      tunnel: w309 -> [w396 w399]
      tunnel: w303 -> [_ w398]
      frame False {
      }
      frame True {
        # "Wchodzą odl. \npołożeń od startu"
        n172 = Enqueue Element(queue=w402, element=w398, error in (no error)=w399) -> (queue out=w401:refnum<queue>, error out=w400:errorcluster)  [unwired: 1 in, 1 out]
      }
    }
    n173 = Wait Until Next ms Multiple(millisecond multiple=u32 40) -> ()  [unwired: 1 out]
    "Prędkości kół" <- w302
  }
  n174 = Release Queue(queue=w12, error in (no error)=w11) -> (error out=w8:errorcluster)  [unwired: 1 in, 2 out]
  n175 = Merge Errors(w8, w3) -> (w7:errorcluster)
  n176 = call <vilib>:"Simple Error Handler.vi"("error in (no error)"=w7) -> ()  [unwired: 4 in, 5 out]
